vi "QA_Plug_In.vi"() -> (5 "Plug in titles":string[](array[string]), 7 "Plug in values":string[](array[string]))   [LabVIEW 2010]
uses:
  Controls/Analysis_type_Enum.ctl
  Globals/Meas_global.vi
  Globals/LDA_meas_global_1.vi
  Globals/Plug_in_data_global.vi
panel:
  out "Number Of samples in T":i32
  out "Number Of samples in V":i32
  out "Number Of samples in U":i32
  out "Analysis type":T1
  out "Current Block No":i32
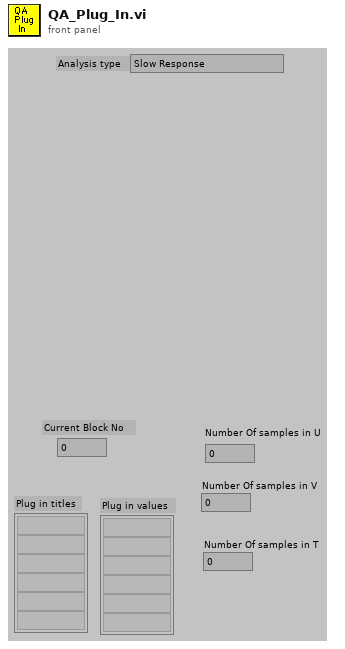
[diagram p1: front panel]
types:
  T1 = typedef "Analysis_type_Enum.ctl" = enum16{"Slow Response", "Fast Response", "Weighted Fast Response", "Fast FID", "Weighted Fast FID", "Cross Wire", "Weighted Cross Wire", "Weighted LDA"}
  T2 = typedef "Analysis_type_cluster.ctl" = cluster{"Analysis type":T1, "Indicies":i32[], "Name":string, "Inst Array":T3, "Info index":i32}
  T3 = typedef "Instrument_Array.ctl" = enum16{"PWA", "LDA", "Analogue"}
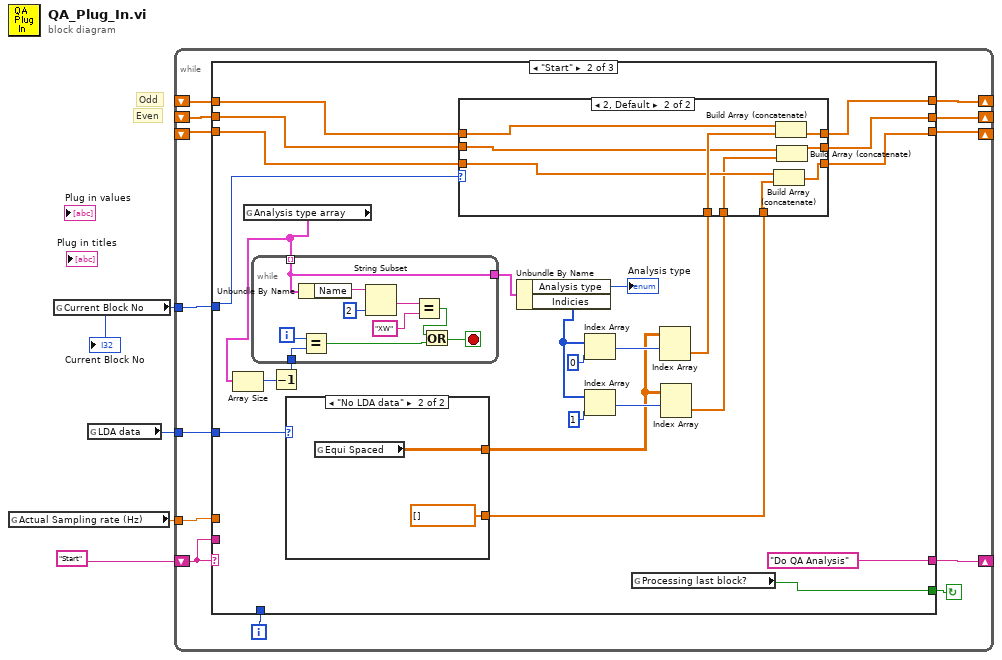
[diagram p0: block diagram]
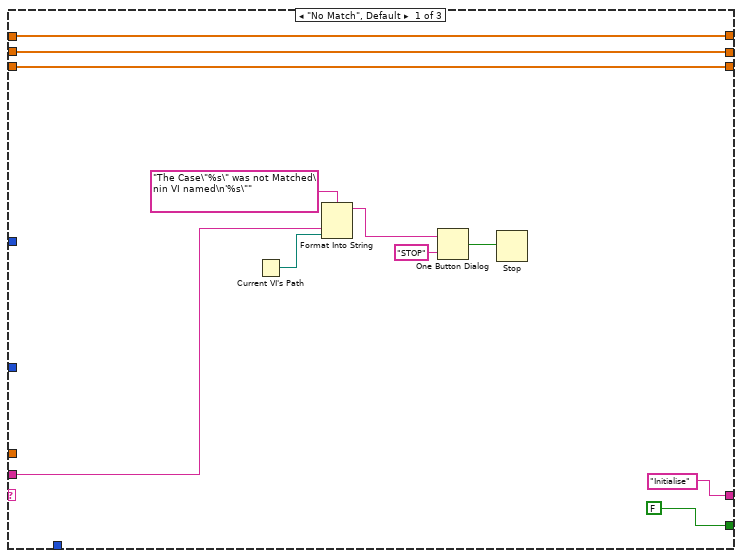
[diagram p2: hidden frame]
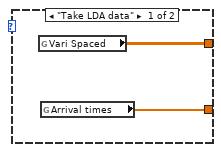
[diagram p3: hidden frame]
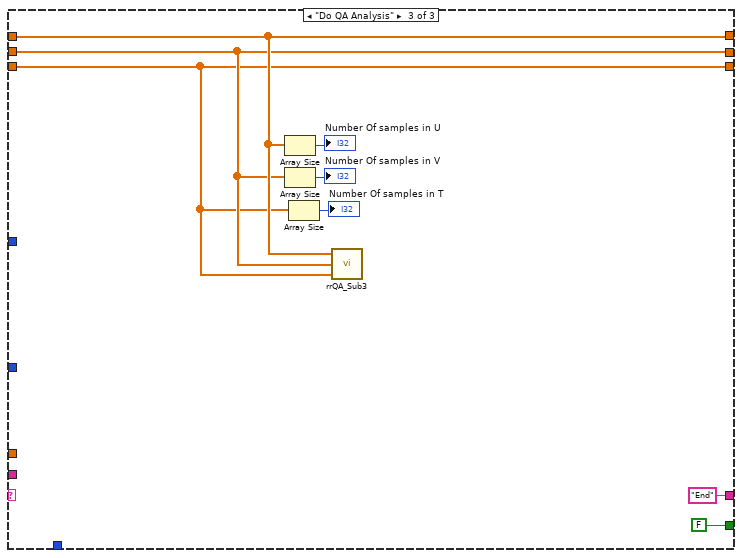
[diagram p5: hidden frame]
diagram:
  # "Even"
  # "Odd"
  n1 = global read "Meas_global.vi" "Actual Sampling rate (Hz)"() -> (w3:dbl)
  n2 = global read "Meas_global.vi" "Current Block No"() -> (w2:i32)
  "Current Block No" <- w2
  n3 = global read "Meas_global.vi" "LDA data"() -> (w1:enum16{"No LDA data", "Take LDA data"})
  n4 = while {
    shift-left: "Start" -> [w15]
    shift-right: [w16] -> _
    shift-right: [w14] -> _
    shift-left: _ -> [w11]
    shift-right: [w13] -> _
    shift-left: _ -> [w12]
    tunnel: w3 -> [w10]
    tunnel: w2 -> [w9]
    shift-right: [w6] -> _
    shift-left: _ -> [w7]
    tunnel: w1 -> [w5]
    i -> [w8]
    stop <- w17 continue-if-true
    n5 = case shown="\"Start\"" w15 {
      tunnel: [FALSE w33 FALSE ("Processing last block?")] -> w17
      tunnel: ["Initialise" "Do QA Analysis" "End"] -> w16
      tunnel: w15 -> [w23 _ _]
      tunnel: [w20 w52 w84] -> w14
      tunnel: [w19 w50 w82] -> w13
      tunnel: w12 -> [w19 w49 w82]
      tunnel: w11 -> [w20 w51 w84]
      tunnel: w10 -> [_ _ _]
      tunnel: w9 -> [_ w45 _]
      tunnel: w8 -> [_ _ _]
      tunnel: w7 -> [w18 w47 w81]
      tunnel: [w18 w48 w81] -> w6
      tunnel: w5 -> [_ w38 _]
      frame "No Match", Default {
        n6 = Current VI's Path() -> (path=w22:path)
        n7 = Format Into String(format string="The Case\"%s\" was not Matched\nin VI named\n'%s\"" ("Format String"), w23, w22) -> (resulting string=w26:string)  [unwired: 2 in, 1 out]
        n8 = One Button Dialog(message=w26, button name ("OK")="STOP") -> (true=w24:bool)
        n9 = Stop(stop? (T)=w24) -> ()
      }
      frame "Start" {
        n10 = global read "Meas_global.vi" "Analysis type array"() -> (w32:T2[])
        n11 = Array Size(array=w32) -> (size(s)=w31:i32)
        n12 = Decrement(x=w31) -> (x-1=w30:i32)
        n13 = while {
          tunnel: w32 -> [w53] mode=indexing
          tunnel: w30 -> [w55]
          tunnel: [w53] -> w29
          i -> [w56]
          stop <- w57 stop-if-true
          n14 = Unbundle By Name(w53) -> ("Name"=w62:string)
          n15 = Equal?(x=w56, y=w55) -> (x = y?=w54:bool)
          n16 = String Subset(string=w62, length (rest)=2 ("length (rest)")) -> (substring=w60:string)  [unwired: 1 out]
          n17 = Equal?(x=w60, y="XW") -> (x = y?=w58:bool)
          n18 = Or(x=w58, y=w54) -> (x .or. y?=w57:bool)
        }
        n19 = case shown="\"No LDA data\"" w38 {
          tunnel: [w63 w66] -> w37
          tunnel: [w64 dbl[] [] ("Arrival times")] -> w34
          frame "Take LDA data" {
            n20 = global read "Plug_in_data_global.vi" "Vari Spaced"() -> (w63:dbl[][])
            n21 = global read "LDA_meas_global_1.vi" "Arrival times"() -> (w64:dbl[])
          }
          frame "No LDA data" {
            n22 = global read "Plug_in_data_global.vi" "Equi Spaced"() -> (w66:dbl[][])
          }
        }
        n23 = Unbundle By Name(w29) -> ("Analysis type"=→"Analysis type":T1, "Indicies"=w43:i32[])
        n24 = Index Array(array=w43, index=0) -> (element=w39:i32)
        n25 = Index Array(array=w43, index=1) -> (element=w40:i32)
        n26 = global read "Meas_global.vi" "Processing last block?"() -> (w33:bool)
        n27 = Index Array(array=w37, index (row)=w39) -> (element=w36:dbl[])  [unwired: 1 in]
        n28 = Index Array(array=w37, index (row)=w40) -> (element=w35:dbl[])  [unwired: 1 in]
        n29 = case shown="2, Default" w45 {
          tunnel: [w69 w76] -> w52
          tunnel: w51 -> [_ w78]
          tunnel: [w68 w70] -> w50
          tunnel: w49 -> [_ w75]
          tunnel: [w67 w71] -> w48
          tunnel: w47 -> [_ w74]
          tunnel: w36 -> [w69 w77]
          tunnel: w35 -> [w68 w73]
          tunnel: w34 -> [w67 w72]
          frame 1 {
          }
          frame 2, Default {
            n30 = Build Array (concatenate)(w74, w72) -> (w71:dbl[])
            n31 = Build Array (concatenate)(w78, w77) -> (w76:dbl[])
            n32 = Build Array (concatenate)(w75, w73) -> (w70:dbl[])
          }
        }
      }
      frame "Do QA Analysis" {
        n33 = Array Size(array=w84) -> (size(s)=→"Number Of samples in U":i32)
        n34 = Array Size(array=w82) -> (size(s)=→"Number Of samples in V":i32)
        n35 = Array Size(array=w81) -> (size(s)=→"Number Of samples in T":i32)
        n36 = call "rrQA_Sub3.vi"("U"=w84, "W"=w82, "T"=w81) -> ()  [unwired: 5 out]
      }
    }
  }
